vi "Permutations of Settings.vi"() -> (3 "Settings Permutations":string[](array[string]))   [LabVIEW 2020]
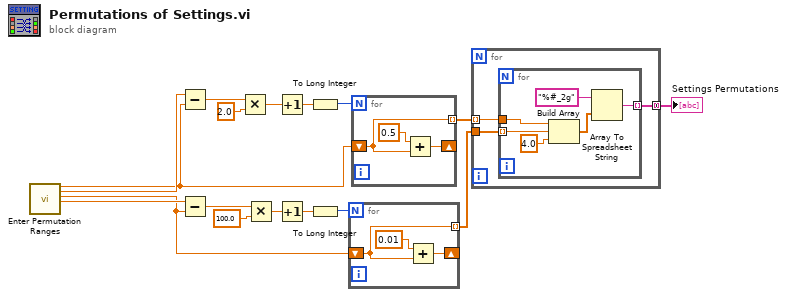
[diagram p0: block diagram]
diagram:
  n1 = call "Enter Permutation Ranges"() -> ("Lower Cutoff Range"=w1:dbl, "Upper Cutoff Range"=w2:dbl, "Lower Threshold Range"=w3:dbl, "Upper Threshold Range"=w4:dbl)  [unwired: 14 in, 2 out]
  n2 = Subtract(x=w2, y=w1) -> (x-y=w7:dbl)
  n3 = Subtract(x=w4, y=w3) -> (x-y=w16:dbl)
  n4 = Multiply(x=w7, y=2.0) -> (x*y=w6:dbl)
  n5 = Multiply(x=w16, y=100.0) -> (x*y=w15:dbl)
  n6 = Increment(x=w6) -> (x+1=w14:dbl)
  n7 = Increment(x=w15) -> (x+1=w13:dbl)
  n8 = To Long Integer(number=w14) -> (32bit integer=w11:i32)
  n9 = To Long Integer(number=w13) -> (32bit integer=w12:i32)
  n10 = for {
    N: w12 -> [_]
    shift-right: [w19] -> _
    shift-left: w3 -> [w20]
    tunnel: [w20] -> w10 mode=indexing
    n11 = Add(x=0.01, y=w20) -> (x+y=w19:dbl)
  }
  n12 = for {
    N: w11 -> [_]
    tunnel: [w21] -> w9 mode=indexing
    shift-right: [w23] -> _
    shift-left: w1 -> [w21]
    n13 = Add(x=0.5, y=w21) -> (x+y=w23:dbl)
  }
  n14 = for {
    tunnel: w10 -> [w26]
    tunnel: w9 -> [w25] mode=indexing
    tunnel: [w24] -> w8 mode=concatenating
    n15 = for {
      tunnel: w26 -> [w32] mode=indexing
      tunnel: w25 -> [w31]
      tunnel: [w30] -> w24 mode=indexing
      n16 = Build Array(w31, w32, 4.0 ("Max Padding")) -> (w28:dbl[])
      n17 = Array To Spreadsheet String(array=w28, 3:"%#_2g" ("format string")) -> (spreadsheet string=w30:string)  [unwired: 1 in]
    }
  }
  "Settings Permutations" <- w8
